vi "Process Messages.vi"(10 "Channels in":refnum<data-value>[](array[refnum]), 11 "Message Queue":refnum<queue>) -> (2 "Channels out":refnum<data-value>[](array[refnum]))   [LabVIEW 2020, in "G-Audio.lvlib" / "Mixer.lvclass"]
uses:
  Mixer.lvclass
  Channel/Channel.lvclass
  Command.ctl
  Message.ctl
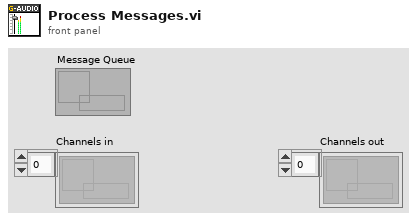
[diagram p1: front panel]
types:
  T1 = typedef "G-Audio.lvlib/Mixer.lvclass/Message.ctl" = cluster{"Command":T2, "Channel":i32, "Payload":variant}
  T2 = typedef "G-Audio.lvlib/Mixer.lvclass/Command.ctl" = enum16{"Channel Stop", "Channel Pause", "Channel Play", "Channel Volume"}
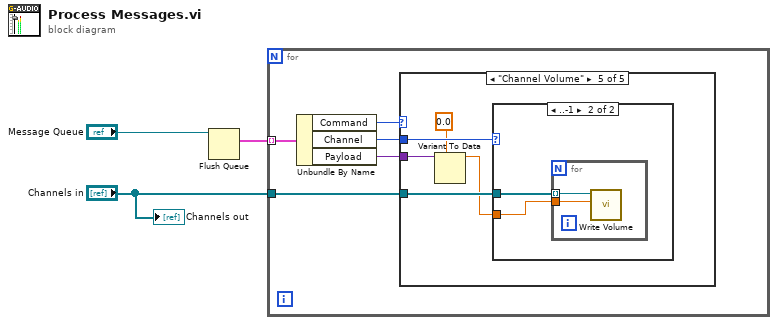
[diagram p0: block diagram]
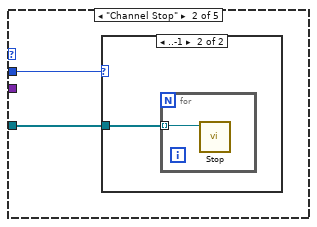
[diagram p3: hidden frame]
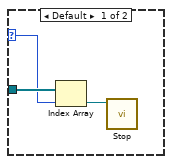
[diagram p4: hidden frame]
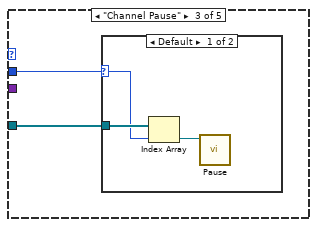
[diagram p5: hidden frame]
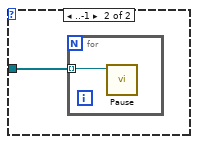
[diagram p6: hidden frame]
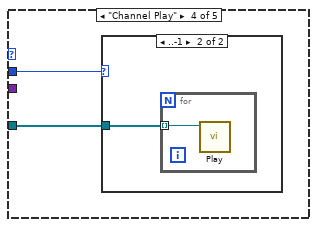
[diagram p7: hidden frame]
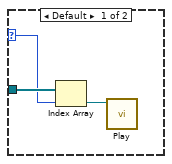
[diagram p8: hidden frame]
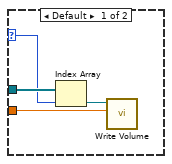
[diagram p9: hidden frame]
diagram:
  n1 = Flush Queue(queue="Message Queue") -> (remaining elements=w2:T1[])  [unwired: 1 in, 2 out]
  n2 = for {
    tunnel: w2 -> [w8] mode=indexing
    tunnel: "Channels in" -> [w6]
    n3 = Unbundle By Name(w8) -> ("Command"=w7:T2, "Channel"=w5:i32, "Payload"=w4:variant)
    n4 = case shown="\"Channel Volume\"" w7 {
      tunnel: w6 -> [_ w10 w17 w24 w34]
      tunnel: w5 -> [_ w9 w16 w23 w33]
      tunnel: w4 -> [_ _ _ _ w32]
      frame Default {
      }
      frame "Channel Stop" {
        n5 = case shown="..-1" w9 {
          selector: w9 -> [w11 _]
          tunnel: w10 -> [w13 w14]
          frame Default {
            n6 = Index Array(array=w13, index=w11) -> (element=w12:refnum<data-value>)
            n7 = call "Stop.vi"("Channel in"=w12) -> ()  [unwired: 9 in, 2 out]
          }
          frame ..-1 {
            n8 = for {
              tunnel: w14 -> [w15] mode=indexing
              n9 = call "Stop.vi"("Channel in"=w15) -> ()  [unwired: 9 in, 2 out]
            }
          }
        }
      }
      frame "Channel Pause" {
        n10 = case shown="Default" w16 {
          selector: w16 -> [w18 _]
          tunnel: w17 -> [w20 w21]
          frame Default {
            n11 = Index Array(array=w20, index=w18) -> (element=w19:refnum<data-value>)
            n12 = call "Pause.vi"("Channel in"=w19) -> ()  [unwired: 9 in, 2 out]
          }
          frame ..-1 {
            n13 = for {
              tunnel: w21 -> [w22] mode=indexing
              n14 = call "Pause.vi"("Channel in"=w22) -> ()  [unwired: 9 in, 2 out]
            }
          }
        }
      }
      frame "Channel Play" {
        n15 = case shown="..-1" w23 {
          selector: w23 -> [w25 _]
          tunnel: w24 -> [w27 w28]
          frame Default {
            n16 = Index Array(array=w27, index=w25) -> (element=w26:refnum<data-value>)
            n17 = call "Play.vi"("Channel in"=w26) -> ()  [unwired: 9 in, 2 out]
          }
          frame ..-1 {
            n18 = for {
              tunnel: w28 -> [w29] mode=indexing
              n19 = call "Play.vi"("Channel in"=w29) -> ()  [unwired: 9 in, 2 out]
            }
          }
        }
      }
      frame "Channel Volume" {
        n20 = Variant To Data(type=sgl 0.0, Variant=w32) -> (data=w30:sgl)  [unwired: 1 in, 1 out]
        n21 = case shown="..-1" w33 {
          selector: w33 -> [w36 _]
          tunnel: w34 -> [w38 w40]
          tunnel: w30 -> [w35 w39]
          frame Default {
            n22 = Index Array(array=w38, index=w36) -> (element=w37:refnum<data-value>)
            n23 = call "Write Volume.vi"("Volume"=w35, "Channel in"=w37) -> ()  [unwired: 8 in, 2 out]
          }
          frame ..-1 {
            n24 = for {
              tunnel: w40 -> [w42] mode=indexing
              tunnel: w39 -> [w41]
              n25 = call "Write Volume.vi"("Volume"=w41, "Channel in"=w42) -> ()  [unwired: 8 in, 2 out]
            }
          }
        }
      }
    }
  }
  "Channels out" <- "Channels in"
